vi "Get Test Numbers.vi"(8 "error in (no error)":errorcluster, 9 "Evaluations In":T1[](array[typedef]) {"Low Limit" format="%#_13g"; "SI Scaling" items=["femto"=-15, "pico"=-12, "nano"=-9, "micro"=-6, "milli"=-3, "percent"=-2, ""=0, "kilo"=3, "mega"=6, "giga"=9, "tera"=12]}, 11 "SPECAN_IQSLOT in":refnum<class "SPECAN_IQSLOT.lvclass">) -> (0 "error out":errorcluster, 1 "Evaluations Out":T1[](array[typedef]) {"Low Limit" format="%#_13g"; "SI Scaling" items=["femto"=-15, "pico"=-12, "nano"=-9, "micro"=-6, "milli"=-3, "percent"=-2, ""=0, "kilo"=3, "mega"=6, "giga"=9, "tera"=12]}, 3 "SPECAN_IQSLOT out":refnum<class "SPECAN_IQSLOT.lvclass">)   [LabVIEW 2018, in "SPECAN_IQSLOT.lvlib" / "SPECAN_IQSLOT.lvclass"]
uses:
  SPECAN_IQSLOT.lvclass
  C:/Sequence Automation/Plugins/Measurement Interface.lvlibp/Measurement Interface.lvclass
  Plugins/TestStand API Tools (TSAT).lvlibp/Evaluation Actions/Includes/Controls/TSAT Evaluation.ctl
  Plugins/TestStand API Tools (TSAT).lvlibp/Evaluation Actions/Includes/Controls/TSAT Eval SI Unit Scaling.ctl
  Plugins/TestStand API Tools (TSAT).lvlibp/Evaluation Actions/Includes/Controls/TSAT Evaluation Type.ctl
  Plugins/Test Number and Bin Generator.lvlibp/Test Number and Bin Generator/Test Number and Bin Generator.lvclass
  Plugins/TestStand API Tools (TSAT).lvlibp/Evaluation Actions/TSAT Evaluation Actions.lvlib
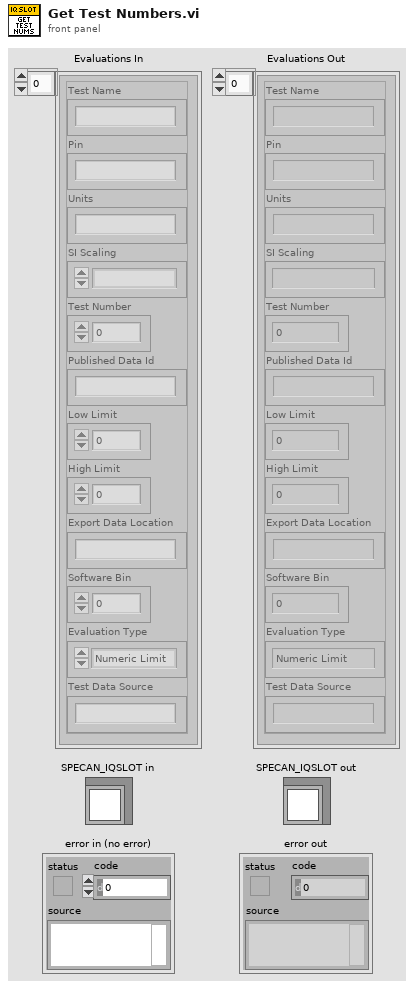
[diagram p1: front panel]
types:
  T1 = typedef "TestStand API Tools (TSAT).lvlibp/TSAT Evaluation Actions.lvlib/TSAT Evaluation.ctl" = cluster{"Test Name":string, "Pin":string, "Units":string, "SI Scaling":T2, "Test Number":i32, "Published Data Id":string, "Low Limit":dbl, "High Limit":dbl, "Export Data Location":string, "Software Bin":i64, "Evaluation Type":T3, "Test Data Source":string}
  T2 = typedef "TestStand API Tools (TSAT).lvlibp/TSAT Evaluation Actions.lvlib/TSAT Eval SI Unit Scaling.ctl" = i16
  T3 = typedef "TestStand API Tools (TSAT).lvlibp/TSAT Evaluation Actions.lvlib/TSAT Evaluation Type.ctl" = enum16{"Numeric Limit", "Pass/Fail", "None"}
  T4 = typedef "Test Number and Bin Generator.lvlibp/Test Number and Bin Generator.lvclass/Session Handle.ctl" = refnum<data-value>
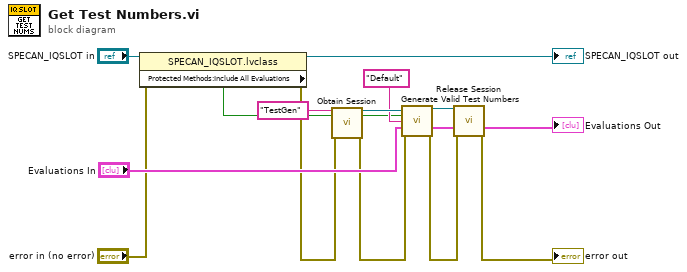
[diagram p0: block diagram]
diagram:
  n1 = property class="SPECAN_IQSLOT.lvclass"(reference="SPECAN_IQSLOT in", error in="error in (no error)") -> (reference out=→"SPECAN_IQSLOT out":refnum<class "SPECAN_IQSLOT.lvclass">, error out=w5:errorcluster, "Protected Methods:Include All Evaluations"=w2:bool)
  n2 = call "Obtain Session.vi"("Session  Name ()"="TestGen", "error in (no error)"=w5) -> ("Session Handle"=w13:T4, "error out"=w8:errorcluster)  [unwired: 12 in]
  n3 = call "Generate Valid Test Numbers.vi"("Session Handle in"=w13, "Include All Evaluations?"=w2, "Test Group"="Default", "Evaluations In"="Evaluations In", "error in (no error)"=w8) -> ("Session Handle out"=w14:T4, "Evaluations Out"=→"Evaluations Out":T1[], "error out"=w7:errorcluster)  [unwired: 8 in]
  n4 = call "Release Session.vi"("Session Handle"=w14, "error in (no error)"=w7) -> ("error out"=→"error out":errorcluster)  [unwired: 13 in]
